vi "Lookup Alarm Info From Alarms Details.vi"(10 "Code":i32, 11 "Alarm Details":T1[](array[typedef])) -> (1 "Severity":i32, 2 "Description":string, 3 "Loop":i32)   [LabVIEW 2015, in "Alarm Handler Actor.lvclass"]
doc: "Searches through the Alarms Details for the alarm specified by <b>Code</b>."
uses:
  Alarm Handler Actor.lvclass
  Alarm Details.ctl
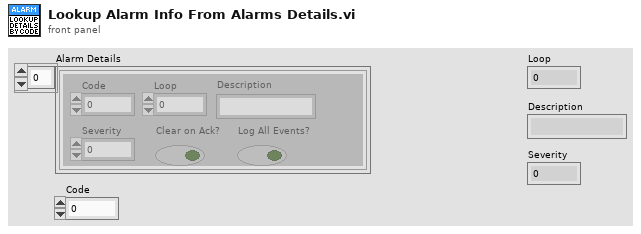
[diagram p1: front panel]
types:
  T1 = typedef "Alarm Handler Actor.lvclass/Alarm Details.ctl" = cluster{"Code":i32, "Loop":i32, "Description":string, "Severity":i32, "Clear on Ack?":bool, "Log All Events?":bool}
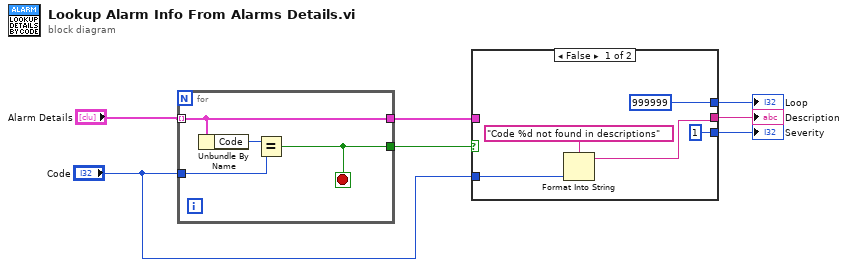
[diagram p0: block diagram]
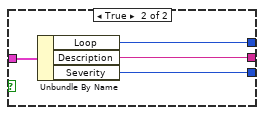
[diagram p2: hidden frame]
diagram:
  n1 = for {
    tunnel: "Alarm Details" -> [w9] mode=indexing
    tunnel: "Code" -> [w10]
    tunnel: [w9] -> w5
    tunnel: [w8] -> w6
    stop <- w8 stop-if-true
    n2 = Unbundle By Name(w9) -> ("Code"=w11:i32)
    n3 = Equal?(x=w11, y=w10) -> (x = y?=w8:bool)
  }
  n4 = case shown="False" w6 {
    tunnel: w5 -> [_ w20]
    tunnel: [999999 ("Loop") w19] -> w4
    tunnel: [w14 w18] -> w3
    tunnel: [1 ("Severity") w17] -> w2
    tunnel: "Code" -> [w13 _]
    frame False {
      n5 = Format Into String(format string="Code %d not found in descriptions", w13) -> (resulting string=w14:string)  [unwired: 2 in, 1 out]
    }
    frame True {
      n6 = Unbundle By Name(w20) -> ("Loop"=w19:i32, "Description"=w18:string, "Severity"=w17:i32)
    }
  }
  "Description" <- w3
  "Loop" <- w4
  "Severity" <- w2
